vi "CODMn校准记录.vi"(8 "错误输入（无错误）":errorcluster, 11 "data in":T1) -> (0 "错误输出":errorcluster)   [LabVIEW 2016, in "斯坦道CODMn新电路板.lvlib"]
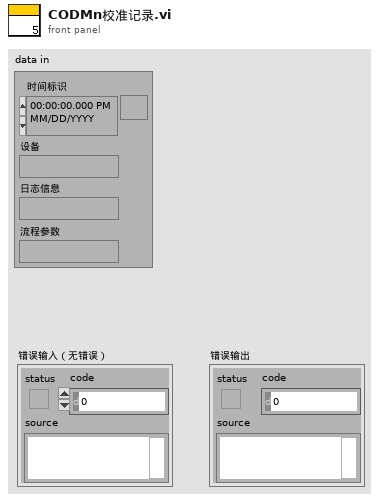
[diagram p1: front panel]
types:
  T1 = cluster{"时间标识":timestamp, "设备":string, "日志信息":string, "流程参数":string}
  T2 = typedef "数据库类型.ctl" = enum16{"Access", "SQLite"}
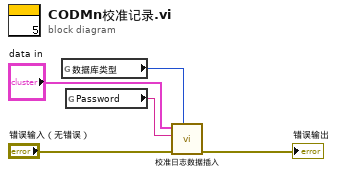
[diagram p0: block diagram]
diagram:
  n1 = global read "CODMn断电保存全局变量.vi" "数据库类型"() -> (w2:T2)
  n2 = global read "CODMn断电保存全局变量.vi" "Password"() -> (w1:string)
  n3 = call "校准日志数据插入.vi"("data"="data in", "Password"=w1, "错误输入（无错误）"="错误输入（无错误）", "数据库类型"=w2) -> ("错误输出"=→"错误输出":errorcluster)  [unwired: 6 in]
